vi "niDTS GNSS GPS Rx RF Test UTIL GNSS to GPS Parameters.vi"(1 "Parameters IN":T1={"GNSS Standard"=enum."GPS", "Frequency (Hz)"=0.0, "Auto Level"=FALSE, "Power (dBm)"=0.0, "External Attenuation (dB)"=0.0, "Measurement Interval (s)"=1000.0, "Pattern"=enum."PN9", "Enable Averaging"=FALSE, "Type Of Averaging"=enum."MEAN", "Number of Averages"=0, "Waveform Name"="", "Enable Traces"=FALSE} {"External Attenuation (dB)" format="%.1g"; "Power (dBm)" format="%.1g"}) -> (0 "Parameters OUT":T2 {"External Attenuation (dB)" format="%.1g"; "Power (dBm)" format="%.1g"})   [LabVIEW 2014, in "niDTS GNSS.lvlib"]
uses:
  niDTS GNSS.lvlib
  Includes/niDTS GNSS GPS Rx RF Test INC Parameters.ctl
  Includes/niDTS GNSS GPS Rx RF Test INC Channel.ctl
  RF Test/Includes/niDTS GNSS RF Test INC Parameters.ctl
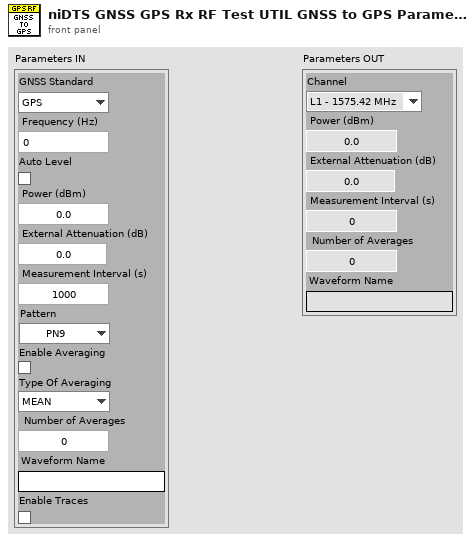
[diagram p1: front panel]
types:
  T1 = typedef "niDTS GNSS.lvlib/niDTS GNSS RF Test INC Parameters.ctl" = cluster{"GNSS Standard":enum16{"GPS", "GLONASS", "Galileo", "Beidou"}, "Frequency (Hz)":dbl, "Auto Level":bool, "Power (dBm)":dbl, "External Attenuation (dB)":dbl, "Measurement Interval (s)":dbl, "Pattern":enum16{"0", "1", "01", "00001111", "PN9"}, "Enable Averaging":bool, "Type Of Averaging":enum16{"MEAN", "MAX", "MIN", "MAXMIN"}, "Number of Averages":i32, "Waveform Name":string, "Enable Traces":bool}
  T2 = typedef "niDTS GNSS.lvlib/niDTS GNSS GPS Rx RF Test INC Parameters.ctl" = cluster{"Channel":T3, "Power (dBm)":dbl, "External Attenuation (dB)":dbl, "Measurement Interval (s)":dbl, "Number of Averages":i32, "Waveform Name":string}
  T3 = typedef "niDTS GNSS.lvlib/niDTS GNSS GPS Rx RF Test INC Channel.ctl" = enum16{"L1 - 1575.42 MHz", "L2 - 1227.60 MHz", "L5 - 1176.45 MHz"}
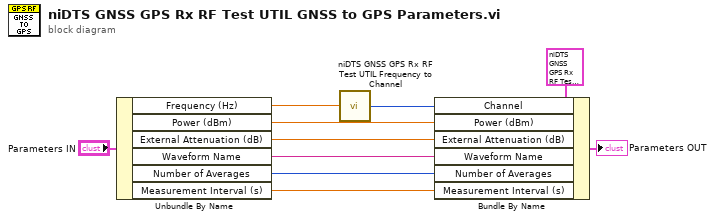
[diagram p0: block diagram]
diagram:
  n1 = Unbundle By Name("Parameters IN") -> ("Frequency (Hz)"=w4:dbl, "Power (dBm)"=w5:dbl, "External Attenuation (dB)"=w6:dbl, "Waveform Name"=w7:string, "Number of Averages"=w2:i32, "Measurement Interval (s)"=w1:dbl)
  n2 = call "niDTS GNSS GPS Rx RF Test UTIL Frequency to Channel.vi"("Frequency (Hz) IN"=w4) -> ("Channel OUT"=w3:T3)
  n3 = Bundle By Name(cluster=T2 {"Channel"=enum."L1 - 1575.42 MHz", "Power (dBm)"=0.0, "External Attenuation (dB)"=0.0, "Measurement Interval (s)"=0.0, "Number of Averages"=0, "Waveform Name"=""} ("Parameters OUT"), "Channel"=w3, "Power (dBm)"=w5, "External Attenuation (dB)"=w6, "Waveform Name"=w7, "Number of Averages"=w2, "Measurement Interval (s)"=w1) -> (→"Parameters OUT":T2)
